vi "Modi Correlation.vi"(2 "d":sgl format="%.2f", 3 "samples":i32, 4 "Rxx in":dbl[](array[numeric]) format="%.2f") -> (0 "n":dbl format="%.2f", 1 "Rxx out":dbl[](array[numeric]) format="%.2f")   [LabVIEW 2010]
doc: "此函数对LabVIEW的相关函数进行修正，将每个相关值除以N-τ。N是LabVIEW的相关函数输出数组的长度，τ是时移的位置。\n Rxx in是LabVIEW的相关函数输出值，Rxx out是修正后的相关值， Samples是取样数，d是输出相关函数首尾截去的百分比。n是截短后的取样数。"
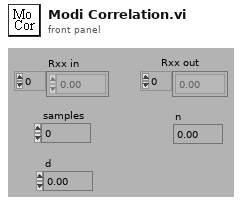
[diagram p1: front panel]
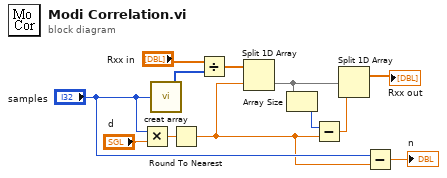
[diagram p0: block diagram]
diagram:
  n1 = Multiply(x="samples", y="d") -> (x*y=w12:sgl)
  n2 = call "creat array.vi"("size"="samples") -> ("array"=w6:i32[])
  n3 = Round To Nearest(number=w12) -> (nearest integer value=w2:sgl)
  n4 = Divide(x="Rxx in", y=w6) -> (x/y=w4:dbl[])
  n5 = Split 1D Array(array=w4, index=w2) -> (second subarray=w9:dbl[])  [unwired: 1 out]
  n6 = Array Size(array=w9) -> (size(s)=w7:i32)
  n7 = Subtract(x=w7, y=w2) -> (x-y=w8:sgl)
  n8 = Split 1D Array(array=w9, index=w8) -> (first subarray=→"Rxx out":dbl[])  [unwired: 1 out]
  n9 = Subtract(x="samples", y=w2) -> (x-y=→"n":sgl)
